vi "G#Object_RegisterClassAttributes.vi"(0 "reference in":refnum<class "G#Object.lvclass">, 1 "static attribute ref":u32, 5 "error in (no error)":errorcluster) -> (14 "reference out":refnum<class "G#Object.lvclass">, 19 "error out":errorcluster)   [LabVIEW 2020, in "G#Object.lvclass"]
doc: "Registers the object to the G# all objects lists. It also sends an event to the debugger and the desktop trace."
uses:
  G#Object.lvclass
  utils/G#Object_ObjectInfoType.ctl
  utils/G#Object_CreateMethod.ctl
  utils/G#Object_EventType.ctl
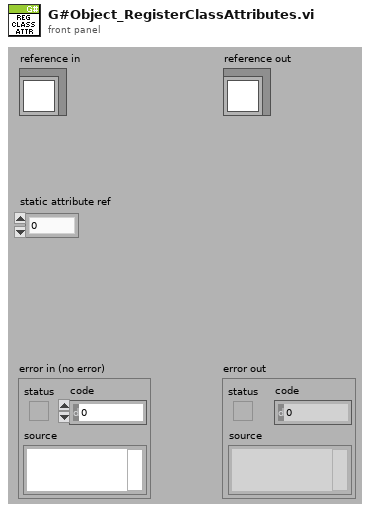
[diagram p1: front panel]
types:
  T1 = typedef "G#Object.lvclass/G#Object_EventType.ctl" = enum16{"Created new", "Looked up existing", "Deleted", "Forced delete", "Not deleted", "Garbage collected", "Cleared", "User", "Error", "External create object", "External create class attributes", "Created class attributes", "Run constructor", "Run constructor done", "Run open method", "Run open method done"}
  T2 = typedef "G#Object.lvclass/G#Object_ObjectInfoType.ctl" = cluster{"ObjectName":string, "ObjectID":u32, "Users":i32, "Counter":bool, "AttributeRefs":u32[], "FullClassName":string, "ClassName":string, "CreateMethod":T3, "GenericDestructorExists":bool, "Owner":string}
  T3 = typedef "G#Object.lvclass/G#Object_CreateMethod.ctl" = enum16{"Create", "Create or look up existing", "Look up existing"}
  T4 = cluster{"full class name":string, "reference in":refnum<class "G#Object.lvclass">}
  T5 = cluster{"full class name":string, "reference in":refnum<class "G#Object.lvclass">}[]
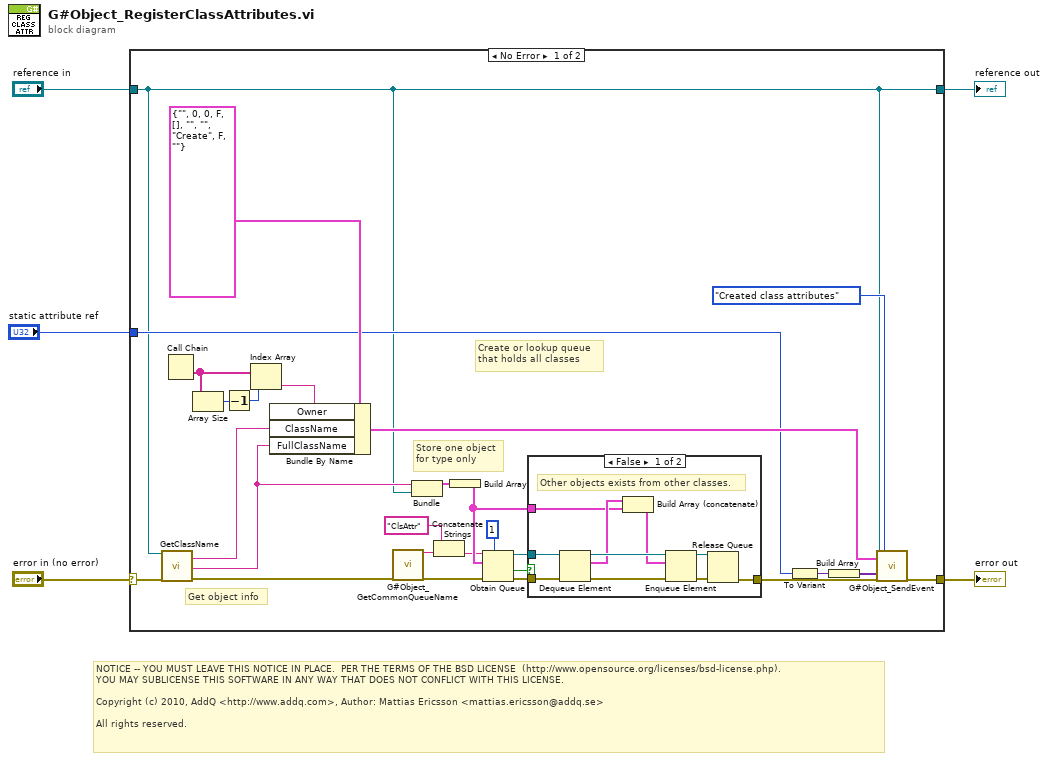
[diagram p0: block diagram]
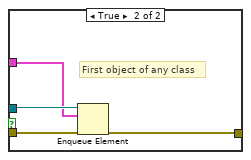
[diagram p2: hidden frame]
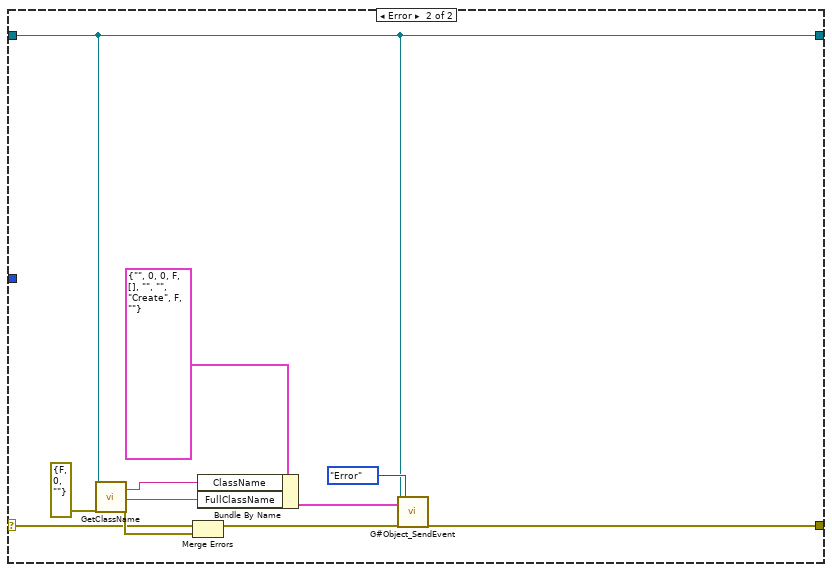
[diagram p3: hidden frame]
diagram:
  # "NOTICE -- YOU MUST LEAVE THIS NOTICE IN PLACE.  PER THE TERMS OF THE BSD LICENSE  (http://www.opensource.org/licenses/bsd-license.php).\nYOU MAY SUBLICENSE THIS SOFTWARE IN ANY WAY THAT DOES NOT CONFLICT WITH THIS LICENSE.\n\nCopyright (c) 2010, AddQ <http://www.addq.com>, Author: Mattias Ericsson <mattias.ericsson@addq.se>\n\nAll rights reserved."
  n1 = case shown="No Error" "error in (no error)" {
    selector: "error in (no error)" -> [w31 w49]
    tunnel: [w32 w57] -> w4
    tunnel: [w8 w47] -> w2
    tunnel: "reference in" -> [w8 w47]
    tunnel: "static attribute ref" -> [w26 _]
    frame No Error {
      # "Store one object\nfor type only"
      # "Create or lookup queue\nthat holds all classes"
      # "Get object info"
      n2 = call-dynamic "GetClassName.vi"("reference in"=w8, "error in (no error)"=w31) -> ("class name"=w28:string, "full class name"=w13:string, "error out"=w7:errorcluster)  [unwired: 13 in, 2 out]
      n3 = Call Chain() -> (call chain=w23:string[])
      n4 = Array Size(array=w23) -> (size(s)=w21:i32)
      n5 = Decrement(x=w21) -> (x-1=w22:i32)
      n6 = Index Array(array=w23, index=w22) -> (element=w20:string)
      n7 = Bundle By Name(cluster=T2 {"ObjectName"="", "ObjectID"=0, "Users"=0, "Counter"=FALSE, "AttributeRefs"=[], "FullClassName"="", "ClassName"="", "CreateMethod"=enum."Create", "GenericDestructorExists"=FALSE, "Owner"=""} ("element"), "Owner"=w20, "ClassName"=w28, "FullClassName"=w13) -> (w29:T2)
      n8 = call "G#Object_GetCommonQueueName.vi"("error in (no error)"=w7) -> ("queue name"=w11:string, "error out"=w12:errorcluster)  [unwired: 17 in]
      n9 = Bundle("full class name"=w13, "reference in"=w8) -> (w14:T4)  [unwired: 1 in]
      n10 = Concatenate Strings("ClsAttr" ("string"), w11) -> (w10:string)
      n11 = Build Array(w14) -> (w16:T5)
      n12 = Obtain Queue(max queue size (-1, unlimited)=1, name (unnamed)=w10, element data type=w16, error in (no error)=w12) -> (queue out=w18:refnum<queue>, created new?=w17:bool, error out=w19:errorcluster)  [unwired: 1 in]
      n13 = case shown="False" w17 {
        tunnel: w19 -> [w37 w46]
        tunnel: [w42 w45] -> w6
        tunnel: w18 -> [w36 w44]
        tunnel: w16 -> [w38 w43]
        frame False {
          # "Other objects exists from other classes."
          n14 = Dequeue Element(queue=w36, error in (no error)=w37) -> (queue out=w41:refnum<queue>, element=w39:T5, error out=w35:errorcluster)  [unwired: 1 in, 1 out]
          n15 = Build Array (concatenate)(w39, w38) -> (w40:T5)
          n16 = Enqueue Element(queue=w41, element=w40, error in (no error)=w35) -> (queue out=w33:refnum<queue>, error out=w34:errorcluster)  [unwired: 1 in, 1 out]
          n17 = Release Queue(queue=w33, error in (no error)=w34) -> (error out=w42:errorcluster)  [unwired: 1 in, 2 out]
        }
        frame True {
          # "First object of any class"
          n18 = Enqueue Element(queue=w44, element=w43, error in (no error)=w46) -> (error out=w45:errorcluster)  [unwired: 1 in, 2 out]
        }
      }
      n19 = To Variant(anything=w26) -> (Variant=w25:variant)
      n20 = Build Array(w25) -> (w24:variant[])
      n21 = call "G#Object_SendEvent.vi"("reference in"=w8, "object info extended"=w29, "parameters"=w24, "error in (no error)"=w6, "G# event type"=G#Object_EventType."Created class attributes" ("G#Event")) -> ("error out"=w32:errorcluster)  [unwired: 14 in]
    }
    frame Error {
      n22 = call-dynamic "GetClassName.vi"("reference in"=w47, "error in (no error)"=errorcluster {"status"=FALSE, "code"=0, "source"=""}) -> ("class name"=w52:string, "full class name"=w51:string, "error out"=w55:errorcluster)  [unwired: 13 in, 2 out]
      n23 = Merge Errors(w49, w55) -> (w48:errorcluster)
      n24 = Bundle By Name(cluster=T2 {"ObjectName"="", "ObjectID"=0, "Users"=0, "Counter"=FALSE, "AttributeRefs"=[], "FullClassName"="", "ClassName"="", "CreateMethod"=enum."Create", "GenericDestructorExists"=FALSE, "Owner"=""}, "ClassName"=w52, "FullClassName"=w51) -> (w50:T2)
      n25 = call "G#Object_SendEvent.vi"("reference in"=w47, "object info extended"=w50, "error in (no error)"=w48, "G# event type"=G#Object_EventType."Error") -> ("error out"=w57:errorcluster)  [unwired: 15 in]
    }
  }
  "error out" <- w4
  "reference out" <- w2
